vi "Teleop.vi"(10 "Match Info":T2={"Autonomous Elapsed Seconds"=0.0, "TeleOp Elapsed Seconds"=50.671, "Disabled Elapsed Seconds"=0.0, "Visited Autonomous"=FALSE, "Visited TeleOp"=TRUE, "Visited Disabled"=FALSE, "Autonomous Settings"={"Autonomous Style"=enum."Independent", "VI Refnum"=refnum}}, 11 "Call Context":T3=enum."Stop") -> ()   [LabVIEW 2017]
doc: "This VI is called for each TeleOp packet received from the DS where the robot is not disabled. It is often used to read from the joysticks and update I/O or to update setpoints for timed control loops. It should complete and return within 20 milliseconds or it may miss DS packets."
uses:
  <vilib>/Rock Robotics/WPI/DriverStation/WPI_DriverStationDerivedRobotMode.ctl
  <vilib>/Rock Robotics/WPI/DriverStation/WPI_DriverStationMatch Info.ctl
  <vilib>/Rock Robotics/Network Tables/NT Read Boolean.vi
  <vilib>/Rock Robotics/Network Tables/NT Read Number.vi
  <vilib>/Rock Robotics/WPI/Utilities/WPI_GetSetVariantRefNum.vi
  <vilib>/Rock Robotics/Network Tables/NT Write Number.vi
  <vilib>/Rock Robotics/Network Tables/NT Write Boolean.vi
  Robot Global Data.vi
  <vilib>/addons/control/pid/pid.llb/PID (DBL).vi
  <vilib>/addons/control/pid/NI_PID_pid.lvlib
panel:
  in  "AntiG 2":dbl=0.3
  in  "Intake Rate":dbl=2.0
  in  "Max Speed":dbl=0.7
  in  "Arm Rate Limiter":dbl=1.0
  in  "Turning Rate Limiter":dbl=4.0
  in  "Throttle Rate Limiter":dbl=4.0
  in  "Intake Speed":dbl=0.3
  in  "Outake Speed":dbl=-0.5
  in  "Throttle Speed Multiplier":dbl=0.35
  in  "Turning Speed Multiplier":dbl=0.6
  in  "Arm Speed Multiplier":dbl=0.3
  out "Waveform Chart":cluster{dbl, dbl}(graph)={-0.0033761270528733234, -0.1}
  in  "PID gains":T1={"proportional gain (Kc)"=1.0, "integral time (Ti, min)"=0.01, "derivative time (Td, min)"=0.0} {"derivative time (Td, min)" format="%.3f"; "integral time (Ti, min)" format="%.3f"; "proportional gain (Kc)" format="%.3f"}
  out "Sample Slider 0":dbl(slide) scale=0.0..5.0
  out "Sample Boolean 0":bool
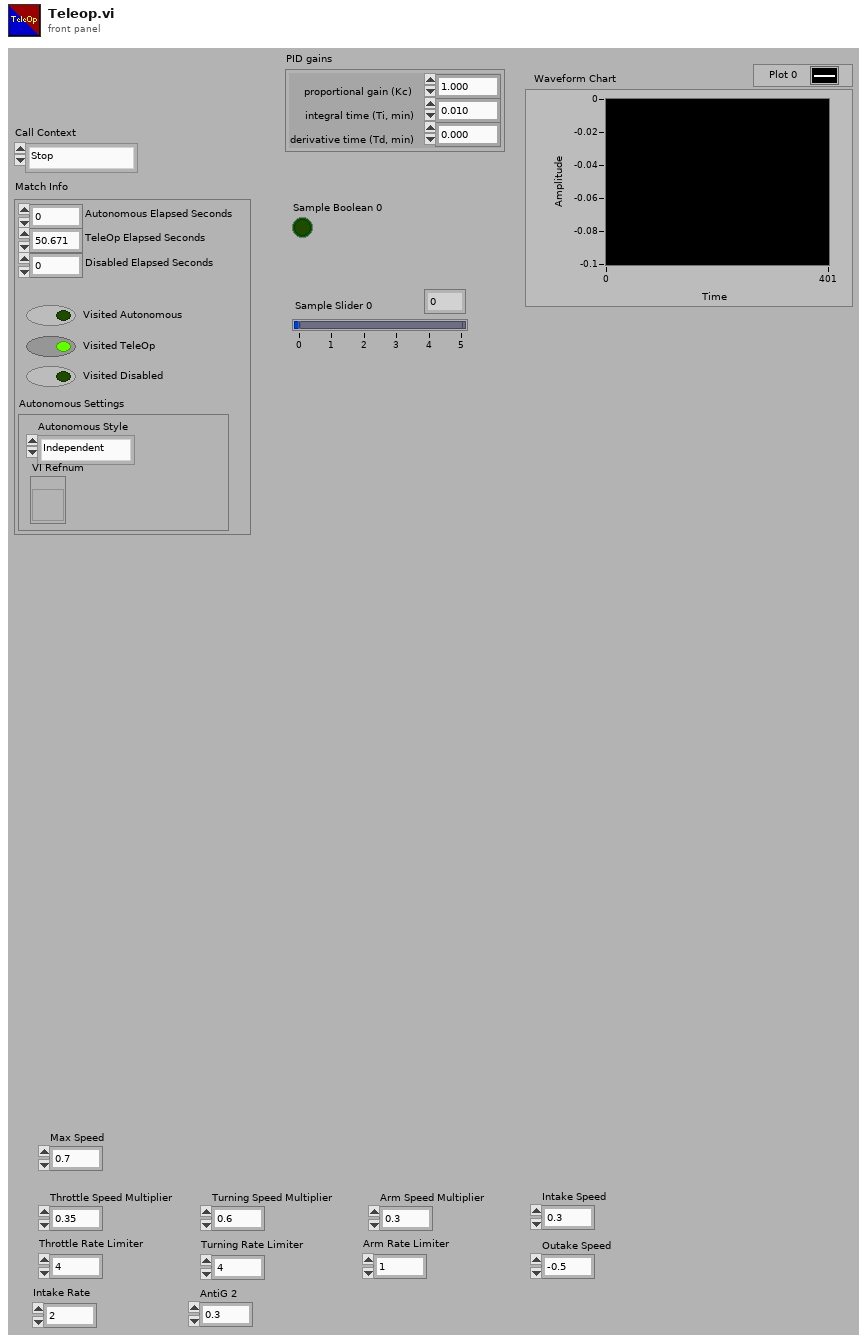
[diagram p1: front panel]
types:
  T1 = cluster{"proportional gain (Kc)":dbl, "integral time (Ti, min)":dbl, "derivative time (Td, min)":dbl}
  T2 = typedef "WPI_DriverStationMatch Info.ctl" = cluster{"Autonomous Elapsed Seconds":dbl, "TeleOp Elapsed Seconds":dbl, "Disabled Elapsed Seconds":dbl, "Visited Autonomous":bool, "Visited TeleOp":bool, "Visited Disabled":bool, "Autonomous Settings":cluster{"Autonomous Style":enum16{"Iterative", "Independent"}, "VI Refnum":refnum<vi>}}
  T3 = typedef "WPI_DriverStationDerivedRobotMode.ctl" = enum16{"Init", "Execute", "Stop"}
  T4 = typedef "WPI_RobotDriveDevRef.ctl" = cluster{"DevStatus":errorcluster, "Motors[]":T5[], "Square Inputs":bool, "Max Output":dbl}
  T5 = typedef "WPI_MotorControlDeviceRef.ctl" = cluster{"DeviceStatus":errorcluster, "Type":T6, "PWM":cluster{"PWM Channel":T7, "DeadBand":T8}, "CAN":cluster{"Device Number":u8, "SetOutput VI Ref":variant, "GetOutput VI Ref":variant, "Enable VI Ref":variant, "Disable VI Ref":variant, "Data":variant}, "Invert":bool, "DIO PWM":cluster{"PWM \"Enable\" Channel":T7, "DIOChannel":T9, "PWM Rate":dbl}}
  T6 = typedef "WPI_MotorControlType.ctl" = enum16{"PWM", "CAN", "DIO PWM"}
  T7 = typedef "FPGA_DIOPWMChannel.ctl" = enum8{"PWM 0", "PWM 1", "PWM 2", "PWM 3", "PWM 4", "PWM 5", "PWM 6", "PWM 7", "PWM 8", "PWM 9", "PWM MXP 0", "PWM MXP 1", "PWM MXP 2", "PWM MXP 3", "PWM MXP 4", "PWM MXP 5", "PWM MXP 6", "PWM MXP 7", "PWM MXP 8", "PWM MXP 9", "Invalid"}
  T8 = typedef "WPI_PWMDeadband.ctl" = cluster{"Name":string, "maxPositivePwm":i32, "minPositivePwm":i32, "centerPwm":i32, "maxNegativePwm":i32, "minNegativePwm":i32, "angularRange":u16}
  T9 = typedef "FPGA_DIOChannel.ctl" = enum8{"DIO 0", "DIO 1", "DIO 2", "DIO 3", "DIO 4", "DIO 5", "DIO 6", "DIO 7", "DIO 8", "DIO 9", "DIO MXP 0", "DIO MXP 1", "DIO MXP 2", "DIO MXP 3", "DIO MXP 4", "DIO MXP 5", "DIO MXP 6", "DIO MXP 7", "DIO MXP 8", "DIO MXP 9", "DIO MXP 10", "DIO MXP 11", "DIO MXP 12", "DIO MXP 13", "DIO MXP 14", "DIO MXP 15", "SPI Port CS1", "SPI Port CS2", "SPI Port CS3", "SPI Port MISO", "SPI Port MOSI", "Invalid"}
  T10 = typedef "WPI_JoystickDevRef.ctl" = cluster{"Device":T11}
  T11 = typedef "WPI_JoystickDeviceEnum.ctl" = enum16{"USB 0", "USB 1", "USB 2", "USB 3", "USB 4", "USB 5"}
  T12 = typedef "WPI_SwitchDevRef.ctl" = cluster{"DevStatus":errorcluster, "DIO Channel":T9, "CntIndex":T13, "Normally Closed":bool}
  T13 = typedef "FPGA_CounterCtrSystemIndex.ctl" = enum8{"Ctr 0", "Ctr 1", "Ctr 2", "Ctr 3", "Ctr 4", "Ctr 5", "Ctr 6", "Ctr 7", "Invalid"}
  T14 = typedef "WPI_PotentiometerDevRef.ctl" = cluster{"DevStatus":errorcluster, "Analog Channel":T15, "Invert Output":bool}
  T15 = typedef "FPGA_AIChannel.ctl" = enum8{"AI 0", "AI 1", "AI 2", "AI 3", "AI MXP 0", "AI MXP 1", "AI MXP 2", "AI MXP 3", "Invalid"}
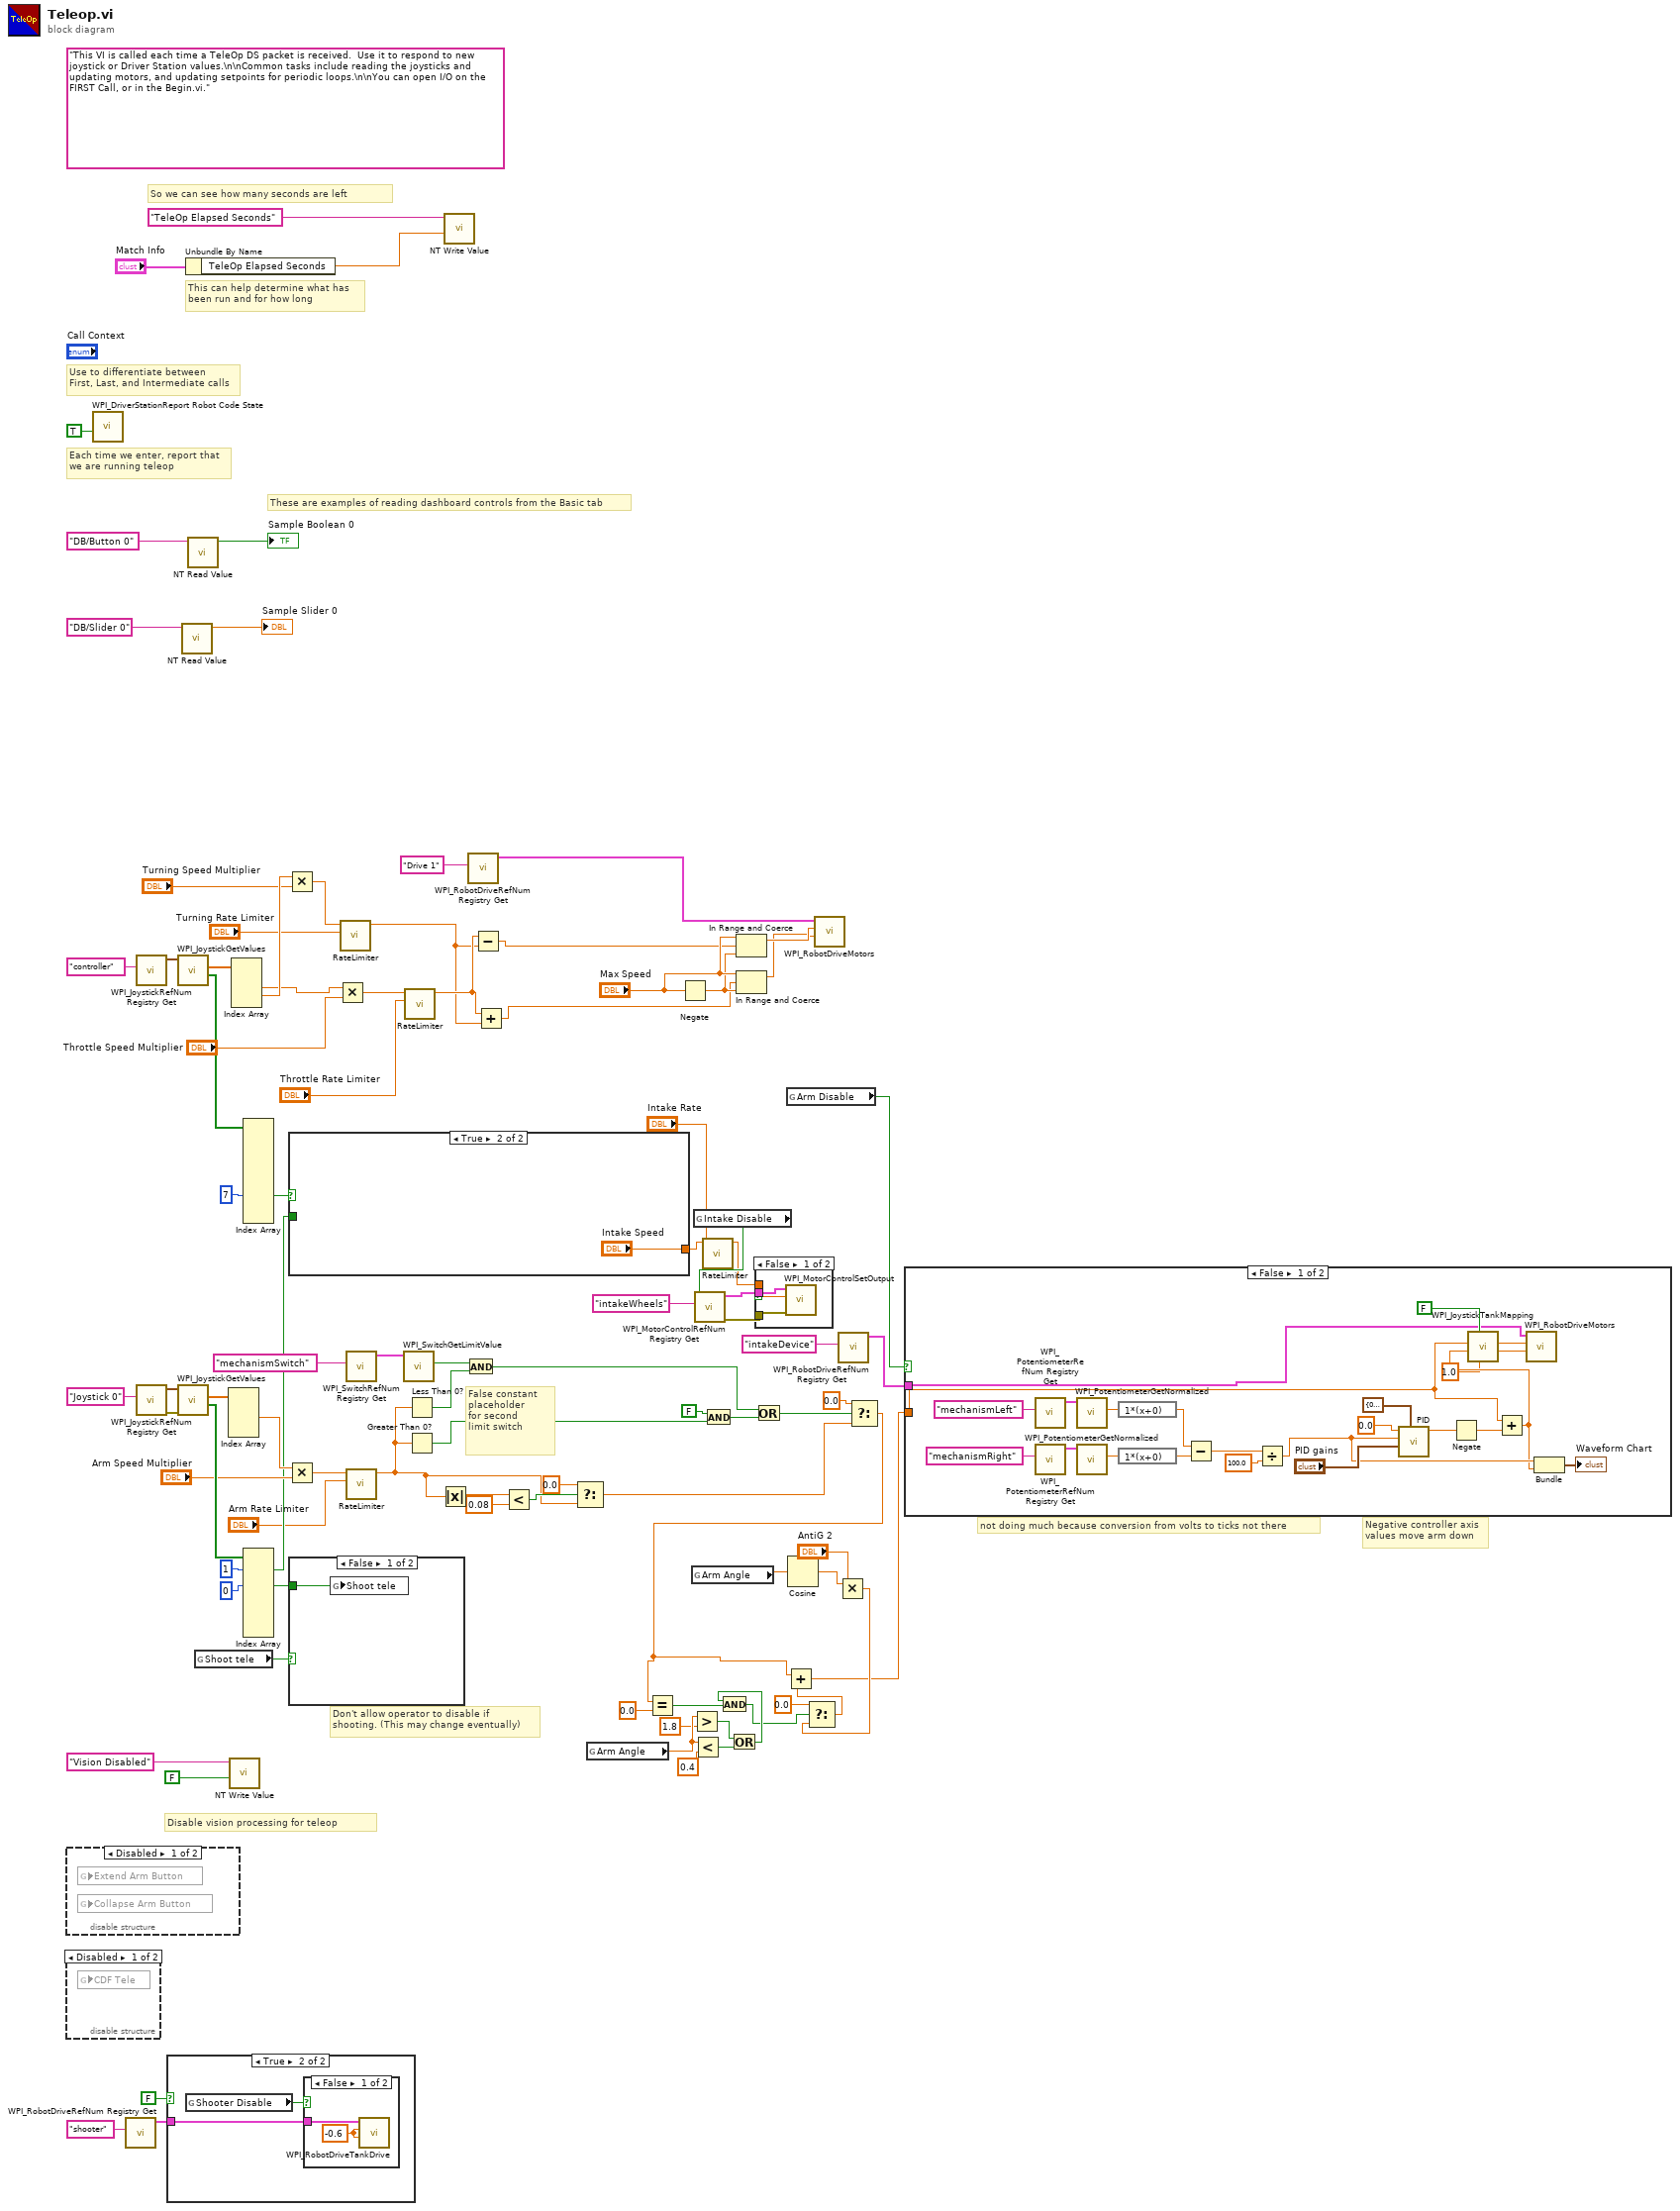
[diagram p0: block diagram]
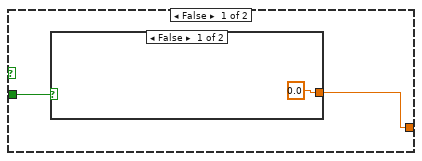
[diagram p3: hidden frame]
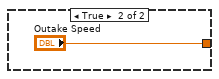
[diagram p4: hidden frame]
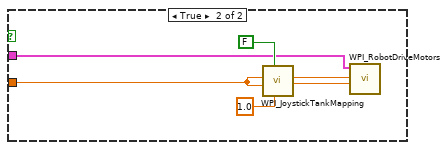
[diagram p9: hidden frame]
diagram:
  (unwired) "This VI is called each time a TeleOp DS packet is received.  Use it to respond to new joystick or Driver Station values.\n\nCommon tasks include reading the joysticks and updating motors, and updating setpoints for periodic loops.\n\nYou can open I/O on the FIRST Call, or in the Begin.vi."
  # "Don't allow operator to disable if\nshooting. (This may change eventually)"
  # "not doing much because conversion from volts to ticks not there"
  # "So we can see how many seconds are left"
  # "False constant \nplaceholder\nfor second \nlimit switch"
  # "Disable vision processing for teleop"
  # "Negative controller axis\nvalues move arm down"
  # "These are examples of reading dashboard controls from the Basic tab"
  # "Each time we enter, report that\nwe are running teleop"
  # "Use to differentiate between\nFirst, Last, and Intermediate calls"
  # "This can help determine what has\nbeen run and for how long"
  n1 = disable-structure shown="Disabled" {
    frame Disabled {
      n2 = global read "Robot Global Data.vi" "Extend Arm Button"() -> ()  [unwired: 1 in]
      n3 = global read "Robot Global Data.vi" "Collapse Arm Button"() -> ()  [unwired: 1 in]
    }
    frame Enabled {
    }
  }
  n4 = disable-structure shown="Disabled" {
    frame Disabled {
      n5 = global read "Robot Global Data.vi" "CDF Tele"() -> ()  [unwired: 1 in]
    }
    frame Enabled {
    }
  }
  n6 = call <vilib>:"WPI_DriverStationReport Robot Code State.vi"("TeleOp"=TRUE ("Autonomous")) -> ()  [unwired: 10 in, 1 out]
  n7 = call <vilib>:"WPI_RobotDriveRefNum Registry Get.vi"("refnum name"="shooter") -> ("RobotDriveDevRef"=w61:T4)  [unwired: 9 in, 1 out]
  n8 = call <vilib>:"WPI_JoystickRefNum Registry Get.vi"("refnum name"="controller") -> ("JoystickDevRef"=w74:T10)  [unwired: 9 in, 1 out]
  n9 = call <vilib>:"WPI_JoystickRefNum Registry Get.vi"("refnum name"="Joystick 0") -> ("error out"=w87:errorcluster, "JoystickDevRef"=w86:T10)  [unwired: 9 in]
  n10 = case shown="True" FALSE {
    tunnel: w61 -> [_ w96]
    frame False {
    }
    frame True {
      n11 = global read "Robot Global Data.vi" "Shooter Disable"() -> (w95:bool)
      n12 = case shown="False" w95 {
        tunnel: w96 -> [w98 _]
        frame False {
          w97 = -0.6 ("Right axis value")
          n13 = call <vilib>:"WPI_RobotDriveTankDrive.vi"("Right axis value"=w97, "Left axis value"=w97, "RobotDriveDevRef"=w98) -> ()  [unwired: 6 in, 3 out]
        }
        frame True {
        }
      }
    }
  }
  n14 = call <vilib>:"WPI_JoystickGetValues.vi"("JoystickDevRef"=w74) -> ("Buttons"=w67:bool[], "Axes"=w73:dbl[])  [unwired: 6 in, 3 out]
  n15 = call <vilib>:"WPI_JoystickGetValues.vi"("error in (no error)"=w87, "JoystickDevRef"=w86) -> ("Buttons"=w88:bool[], "Axes"=w84:dbl[])  [unwired: 5 in, 3 out]
  n16 = call-poly <vilib>:"NT Read Value.vi"("Name"="DB/Slider 0" ("refnum name")) -> ("Numeric"=→"Sample Slider 0":dbl)  [unwired: 9 in, 1 out]
  n17 = Unbundle By Name("Match Info") -> ("TeleOp Elapsed Seconds"=w77:dbl)
  n18 = call-poly <vilib>:"NT Read Value.vi"("Name"="DB/Button 0" ("refnum name")) -> ("Boolean"=→"Sample Boolean 0":bool)  [unwired: 9 in, 1 out]
  n19 = global read "Robot Global Data.vi" "Shoot tele"() -> (w65:bool)
  n20 = Index Array(array=w84) -> (element #2=w59:dbl)  [unwired: 4 in, 3 out]
  n21 = call-poly <vilib>:"NT Write Value.vi"("Boolean"=FALSE, "Name"="Vision Disabled") -> ()  [unwired: 9 in, 1 out]
  n22 = Index Array(array=w73) -> (element #2=w34:dbl, element #3=w56:dbl)  [unwired: 4 in, 2 out]
  n23 = Index Array(array=w67, index #8=7 ("index")) -> (element #8=w51:bool)  [unwired: 10 in, 10 out]
  n24 = Index Array(array=w88, index #1=1 ("index"), index #3=0 ("index")) -> (element #1=w48:bool, element #3=w60:bool)  [unwired: 7 in, 7 out]
  n25 = Multiply(x=w56, y="Turning Speed Multiplier") -> (x*y=w45:dbl)
  n26 = Multiply(x=w59, y="Arm Speed Multiplier") -> (x*y=w43:dbl)
  n27 = case shown="True" w51 {
    tunnel: w48 -> [w100 _]
    tunnel: [w99 "Intake Speed"] -> w30
    frame False {
      n28 = case shown="False" w100 {
        tunnel: [0.0 ("Outake Speed") "Outake Speed"] -> w99
        frame False {
        }
        frame True {
        }
      }
    }
    frame True {
    }
  }
  n29 = case shown="False" w65 {
    tunnel: w60 -> [w104 _]
    frame False {
      n30 = global write "Robot Global Data.vi" "Shoot tele"(w104) -> ()
    }
    frame True {
    }
  }
  n31 = Multiply(x=w34, y="Throttle Speed Multiplier") -> (x*y=w47:dbl)
  n32 = call "RateLimiter.vi"("Max dx/dt"="Turning Rate Limiter", "Input"=w45) -> ("Output"=w2:dbl)  [unwired: 9 in]
  n33 = call <vilib>:"WPI_SwitchRefNum Registry Get.vi"("refnum name"="mechanismSwitch") -> ("SwitchDevRef"=w80:T12)  [unwired: 9 in, 1 out]
  n34 = call "RateLimiter.vi"("Max dx/dt"="Arm Rate Limiter", "Input"=w43) -> ("Output"=w22:dbl)  [unwired: 9 in]
  n35 = call <vilib>:"WPI_SwitchGetLimitValue.vi"("SwitchDevRef"=w80) -> ("Switch Pressed"=w79:bool)  [unwired: 8 in, 2 out]
  n36 = call "RateLimiter.vi"("Max dx/dt"="Throttle Rate Limiter", "Input"=w47) -> ("Output"=w3:dbl)  [unwired: 9 in]
  n37 = Less Than 0?(x=w22) -> (x < 0?=w78:bool)
  n38 = Greater Than 0?(x=w22) -> (x > 0?=w72:bool)
  n39 = Absolute Value(x=w22) -> (abs(x)=w25:dbl)
  n40 = call-poly <vilib>:"NT Write Value.vi"("Numeric"=w77, "Name"="TeleOp Elapsed Seconds") -> ()  [unwired: 9 in, 1 out]
  n41 = And(x=w79, y=w78) -> (x .and. y?=w70:bool)
  n42 = call <vilib>:"WPI_RobotDriveRefNum Registry Get.vi"("refnum name"="Drive 1") -> ("RobotDriveDevRef"=w33:T4)  [unwired: 9 in, 1 out]
  n43 = Subtract(x=w3, y=w2) -> (x-y=w4:dbl)
  n44 = Add(x=w3, y=w2) -> (x+y=w1:dbl)
  n45 = Less?(x=w25, y=0.08) -> (x < y?=w26:bool)
  n46 = Select(t=0.0, s=w26, f=w22) -> (s? t:f=w23:dbl)
  n47 = global read "Robot Global Data.vi" "Arm Angle"() -> (w10:dbl)
  n48 = Negate(x="Max Speed") -> (-x=w38:dbl)
  n49 = global read "Robot Global Data.vi" "Arm Angle"() -> (w21:dbl)
  n50 = Greater?(x=w10, y=1.8) -> (0:w8:bool)
  n51 = Less?(x=w10, y=0.4) -> (x < y?=w11:bool)
  n52 = global read "Robot Global Data.vi" "Intake Disable"() -> (w35:bool)
  n53 = call <vilib>:"WPI_MotorControlRefNum Registry Get.vi"("refnum name"="intakeWheels") -> ("error out"=w49:errorcluster, "MotorControlDevRef"=w50:T5)  [unwired: 9 in]
  n54 = call "RateLimiter.vi"("Max dx/dt"="Intake Rate", "Input"=w30) -> ("Output"=w29:dbl)  [unwired: 9 in]
  n55 = And(x=FALSE, y=w72) -> (x .and. y?=w71:bool)
  n56 = Or(x=w8, y=w11) -> (x .or. y?=w6:bool)
  n57 = In Range and Coerce(upper limit="Max Speed", x=w4, lower limit=w38) -> (coerced(x)=w32:dbl)  [unwired: 1 out]
  n58 = In Range and Coerce(upper limit="Max Speed", x=w1, lower limit=w38) -> (coerced(x)=w31:dbl)  [unwired: 1 out]
  n59 = Or(x=w70, y=w71) -> (x .or. y?=w57:bool)
  n60 = case shown="False" w35 {
    tunnel: w50 -> [w107 _]
    tunnel: w49 -> [w106 _]
    tunnel: w29 -> [w105 _]
    frame False {
      n61 = call <vilib>:"WPI_MotorControlSetOutput.vi"("error in (no error)"=w106, "Output"=w105, "MotorControlDevRef"=w107) -> ()  [unwired: 6 in, 3 out]
    }
    frame True {
    }
  }
  n62 = global read "Robot Global Data.vi" "Arm Disable"() -> (w64:bool)
  n63 = Cosine(x=w21) -> (cos(x)=w20:dbl)
  n64 = call <vilib>:"WPI_RobotDriveMotors.vi"("RightSpeed"=w31, "LeftSpeed"=w32, "RobotDriveDevRef"=w33) -> ()  [unwired: 1 in, 8 out]
  n65 = Multiply(x=w20, y="AntiG 2") -> (x*y=w17:dbl)
  n66 = call <vilib>:"WPI_RobotDriveRefNum Registry Get.vi"("refnum name"="intakeDevice") -> ("RobotDriveDevRef"=w82:T4)  [unwired: 9 in, 1 out]
  n67 = Select(t=0.0, s=w57, f=w23) -> (s? t:f=w14:dbl)
  n68 = Equal?(x=w14, y=0.0) -> (x = y?=w7:bool)
  n69 = And(x=w6, y=w7) -> (x .and. y?=w5:bool)
  n70 = Select(t=0.0, s=w5, f=w17) -> (s? t:f=w16:dbl)
  n71 = Add(x=w14, y=w16) -> (x+y=w13:dbl)
  n72 = case shown="False" w64 {
    tunnel: w82 -> [w109 w134]
    tunnel: w13 -> [w114 w133]
    frame False {
      n73 = call <vilib>:"WPI_PotentiometerRefNum Registry Get.vi"("refnum name"="mechanismLeft") -> ("PotDevRef"=w124:T14)  [unwired: 9 in, 1 out]
      n74 = call <vilib>:"WPI_PotentiometerRefNum Registry Get.vi"("refnum name"="mechanismRight") -> ("PotDevRef"=w125:T14)  [unwired: 9 in, 1 out]
      n75 = call <vilib>:"WPI_PotentiometerGetNormalized.vi"("PotDevRef"=w124) -> ("Normalized Value"=w123:dbl)  [unwired: 8 in, 2 out]
      n76 = call <vilib>:"WPI_PotentiometerGetNormalized.vi"("PotDevRef"=w125) -> ("Normalized Value"=w126:dbl)  [unwired: 8 in, 2 out]
      n77 = expression code="1*(x+0)"(w123) -> (w128:dbl)
      n78 = expression code="1*(x+0)"(w126) -> (w129:dbl)
      n79 = Subtract(x=w128, y=w129) -> (x-y=w121:dbl)
      n80 = Divide(x=w121, y=100.0) -> (x/y=w118:dbl)
      n81 = call-poly <vilib>:"PID.vi"("output range"=cluster{"output high":dbl, "output low":dbl} {"output high"=0.1, "output low"=-0.1}, "PID gains"="PID gains", "process variable"=w118, "setpoint"=0.0) -> ("output"=w116:dbl)  [unwired: 6 in, 1 out]
      n82 = Negate(x=w116) -> (-x=w115:dbl)
      n83 = Add(x=w114, y=w115) -> (x+y=w113:dbl)
      n84 = call <vilib>:"WPI_JoystickTankMapping.vi"("Max Output"=1.0, "Square Inputs"=FALSE, "Right axis value"=w113, "Left axis value"=w114) -> ("Right Motor Value"=w110:dbl, "Left Motor Value"=w111:dbl)  [unwired: 6 in]
      n85 = call <vilib>:"WPI_RobotDriveMotors.vi"("RightSpeed"=w110, "LeftSpeed"=w111, "RobotDriveDevRef"=w109) -> ()  [unwired: 1 in, 8 out]
      n86 = Bundle(w118, w113) -> (→"Waveform Chart":cluster{dbl, dbl})  [unwired: 1 in]
    }
    frame True {
      n87 = call <vilib>:"WPI_JoystickTankMapping.vi"("Max Output"=1.0, "Square Inputs"=FALSE, "Right axis value"=w133, "Left axis value"=w133) -> ("Right Motor Value"=w135:dbl, "Left Motor Value"=w136:dbl)  [unwired: 6 in]
      n88 = call <vilib>:"WPI_RobotDriveMotors.vi"("RightSpeed"=w135, "LeftSpeed"=w136, "RobotDriveDevRef"=w134) -> ()  [unwired: 1 in, 8 out]
    }
  }
